vi "HFRR ADV v10.vi"() -> ()   [LabVIEW 2025] (continued)
                  n3633 = property on="Select Printer 3" class="DigNum (strict)"("Caption.Text"=w4909) -> ()  [unwired: 2 in, 2 out]
                }
                frame 116 {
                  n3634 = property on="Print" class="Bool (strict)"("Boolean Text.Text"=w4910) -> ()  [unwired: 2 in, 2 out]
                }
                frame 117 {
                  "String 41" <- w4911
                }
                frame 118 {
                  n3635 = property on="tested by" class="Str"("Caption.Text"=w4912) -> ()  [unwired: 2 in, 2 out]
                }
                frame 119 {
                }
                frame 120 {
                  n3636 = property on="Export" class="Bool (strict)"("Boolean Text.Text"=w4913) -> ()  [unwired: 2 in, 2 out]
                }
                frame 121 {
                  n3637 = property on="TEMP INTERCEPT:" class="DigNum (strict)"("Caption.Text"=w4914) -> ()  [unwired: 2 in, 2 out]
                }
                frame 122 {
                  n3638 = property on="AIR TEMP INTERCEPT:" class="DigNum (strict)"("Caption.Text"=w4915) -> ()  [unwired: 2 in, 2 out]
                }
                frame 123 {
                  n3639 = property on="Select File Type" class="Enum (strict)"("Caption.Text"=w4916) -> ()  [unwired: 2 in, 2 out]
                }
                frame 124 {
                  n3640 = property on="s.NO" class="Str"("Caption.Text"=w4917) -> ()  [unwired: 2 in, 2 out]
                  "String 45" <- w4917
                }
                frame 125 {
                  n3641 = property on="trip1 8" class="Bool (strict)"("Boolean Text.Text"=w4918) -> ()  [unwired: 2 in, 2 out]
                }
                frame 126, Default {
                }
              }
            }
          }
          frame #1 {
            w4926 = TRUE ("Visible")
            n3642 = local read "S 91"() -> (w4943:string)
            n3643 = local read "S 90"() -> (w4942:string)
            n3644 = local read "S 88"() -> (w4941:string)
            n3645 = property on="Threshold" class="DigNum (strict)"("Caption.Text"=w4943) -> ()  [unwired: 2 in, 2 out]
            n3646 = property on="File Path" class="Path"("Caption.Text"=w4942) -> ()  [unwired: 2 in, 2 out]
            n3647 = property on="SrvM CP" class="Bool (strict)"("Boolean Text.Text"=w4941) -> ()  [unwired: 2 in, 2 out]
            n3648 = local read "S 71"() -> (w4936:string)
            n3649 = local read "S 86"() -> (w4938:string)
            n3650 = local read "S 85"() -> (w4939:string)
            n3651 = local read "S 87"() -> (w4937:string)
            n3652 = local read "S 84"() -> (w4940:string)
            n3653 = local read "S 103"() -> (w4925:string)
            n3654 = local read "S 104"() -> (w4924:string)
            n3655 = property on="ENTER THE NEW PASSWORD" class="Str"("Caption.Text"=w4937) -> ()  [unwired: 2 in, 2 out]
            n3656 = property on="Password" class="Str"("Caption.Text"=w4939) -> ()  [unwired: 2 in, 2 out]
            n3657 = property on="ENTER CURRENT PASSWORD" class="Str"("Caption.Text"=w4938) -> ()  [unwired: 2 in, 2 out]
            n3658 = property on="EDIT" class="Bool (strict)"("Boolean Text.Text"=w4936) -> ()  [unwired: 2 in, 2 out]
            n3659 = property on="SAVE" class="Bool (strict)"("Boolean Text.Text"=w4940) -> ()  [unwired: 2 in, 2 out]
            n3660 = Build Array(w4925, w4924) -> (w4923:string[])
            n3661 = property on="Heater Button" class="Bool (strict)"("Strings [4]"=w4923) -> ()  [unwired: 2 in, 2 out]
            n3662 = property on="CH-HUMIDITY WET" class="DigNum (strict)"("Caption.Size to Text?"=w4926) -> ()  [unwired: 2 in, 2 out]
            n3663 = property on="CH-HUMIDITY DRY" class="DigNum (strict)"("Caption.Size to Text?"=w4926) -> ()  [unwired: 2 in, 2 out]
            n3664 = property on="CH-POWER -" class="DigNum (strict)"("Caption.Size to Text?"=w4926) -> ()  [unwired: 2 in, 2 out]
            n3665 = property on="CH-HEATER" class="DigNum (strict)"("Caption.Size to Text?"=w4926) -> ()  [unwired: 2 in, 2 out]
            n3666 = property on="CH-POWER +" class="DigNum (strict)"("Caption.Size to Text?"=w4926) -> ()  [unwired: 2 in, 2 out]
            n3667 = local read "S 92"() -> (w4935:string)
            n3668 = local read "S 93"() -> (w4934:string)
            n3669 = local read "S 105"() -> (w4921:string)
            n3670 = local read "S 106"() -> (w4920:string)
            n3671 = Build Array(w4935, w4934) -> ()  [unwired: 1 out]
            n3672 = Build Array(w4921, w4920) -> (w4922:string[])
            n3673 = local read "S 95"() -> (w4932:string)
            n3674 = local read "S 94"() -> (w4933:string)
            n3675 = local read "bs"() -> (w4948:string)
            n3676 = local read "as"() -> (w4949:string)
            n3677 = property on="Humidity" class="Bool (strict)"("Strings [4]"=w4922) -> ()  [unwired: 2 in, 2 out]
            n3678 = Concatenate Strings(w4948, "\r", w4949) -> ()  [unwired: 1 out]
            n3679 = property on="STROKE GAIN :" class="DigNum (strict)"("Caption.Text"=w4932) -> ()  [unwired: 2 in, 2 out]
            n3680 = property on="DISPLACEMENT :" class="DigNum (strict)"("Caption.Text"=w4933) -> ()  [unwired: 2 in, 2 out]
            n3681 = property on="Rh After" class="DigNum (strict)"("Caption.Size to Text?"=TRUE ("Caption.Size to Text")) -> ()  [unwired: 2 in, 2 out]
            n3682 = local read "S 48"() -> (w4972:string)
            n3683 = local read "S 50"() -> (w4970:string)
            n3684 = local read "S 51"() -> (w4969:string)
            n3685 = local read "S 49"() -> (w4971:string)
            n3686 = local read "S 52"() -> (w4968:string)
            n3687 = local read "as"() -> (w4953:string)
            n3688 = local read "bs"() -> (w4954:string)
            n3689 = local read "S 56"() -> (w4967:string)
            n3690 = local read "S 57"() -> (w4966:string)
            n3691 = local read "S 58"() -> (w4965:string)
            n3692 = local read "S 59"() -> (w4964:string)
            n3693 = property on="OPEN" class="Bool (strict)"("Boolean Text.Text"=w4968) -> ()  [unwired: 2 in, 2 out]
            n3694 = property on="OPEN 1" class="Bool (strict)"("Boolean Text.Text"=w4972) -> ()  [unwired: 2 in, 2 out]
            n3695 = property on="OPEN 2" class="Bool (strict)"("Boolean Text.Text"=w4971) -> ()  [unwired: 2 in, 2 out]
            n3696 = property on="OPEN 3" class="Bool (strict)"("Boolean Text.Text"=w4970) -> ()  [unwired: 2 in, 2 out]
            n3697 = property on="OPEN 4" class="Bool (strict)"("Boolean Text.Text"=w4969) -> ()  [unwired: 2 in, 2 out]
            n3698 = Concatenate Strings(w4954, "\r", w4953) -> ()  [unwired: 1 out]
            n3699 = local read "S 102"() -> (w4927:string)
            n3700 = property on="КОФ1" class="DigNum (strict)"("Caption.Text"=w4967) -> ()  [unwired: 2 in, 2 out]
            n3701 = local read "S 98"() -> (w4931:string)
            n3702 = local read "S 99"() -> (w4930:string)
            n3703 = local read "S 100"() -> (w4929:string)
            n3704 = local read "S 101"() -> (w4928:string)
            n3705 = property on="КОФ2" class="DigNum (strict)"("Caption.Text"=w4966) -> ()  [unwired: 2 in, 2 out]
            n3706 = property on="КОФ3" class="DigNum (strict)"("Caption.Text"=w4965) -> ()  [unwired: 2 in, 2 out]
            n3707 = property on="КОФ4" class="DigNum (strict)"("Caption.Text"=w4964) -> ()  [unwired: 2 in, 2 out]
            n3708 = local read "bs"() -> (w4952:string)
            n3709 = local read "as"() -> (w4951:string)
            n3710 = property on="CH-POWER +" class="DigNum (strict)"("Caption.Text"=w4931) -> ()  [unwired: 2 in, 2 out]
            n3711 = property on="CH-POWER -" class="DigNum (strict)"("Caption.Text"=w4930) -> ()  [unwired: 2 in, 2 out]
            n3712 = property on="CH-HEATER" class="DigNum (strict)"("Caption.Text"=w4929) -> ()  [unwired: 2 in, 2 out]
            n3713 = property on="CH-HUMIDITY DRY" class="DigNum (strict)"("Caption.Text"=w4928) -> ()  [unwired: 2 in, 2 out]
            n3714 = property on="CH-HUMIDITY WET" class="DigNum (strict)"("Caption.Text"=w4927) -> ()  [unwired: 2 in, 2 out]
            n3715 = local read "S 60"() -> (w4963:string)
            n3716 = local read "S 54"() -> (w4973:string)
            n3717 = Concatenate Strings(w4952, "\r", w4951) -> ()  [unwired: 1 out]
            n3718 = Concatenate Strings(w4973, w4963) -> ()  [unwired: 1 out]
            n3719 = local read "S 77"() -> (→"String 43":string)
            n3720 = local read "S 76"() -> (w4946:string)
            n3721 = local read "S 78"() -> (w4945:string)
            n3722 = local read "S 71"() -> (w4957:string)
            n3723 = local read "S 66"() -> (w4962:string)
            n3724 = local read "S 67"() -> (w4961:string)
            n3725 = local read "S 68"() -> (w4960:string)
            n3726 = local read "S 69"() -> (w4959:string)
            n3727 = local read "S 70"() -> (w4958:string)
            n3728 = property on="AIR TEMP" class="DigNum (strict)"("Caption.Text"=w4945) -> ()  [unwired: 2 in, 2 out]
            n3729 = property on="Set Strk" class="DigNum (strict)"("Caption.Text"=w4946) -> ()  [unwired: 2 in, 2 out]
            n3730 = property on="FRIC. FORCE :" class="DigNum (strict)"("Caption.Text"=w4962) -> ()  [unwired: 2 in, 2 out]
            n3731 = property on="TEMPERATURE :" class="DigNum (strict)"("Caption.Text"=w4961) -> ()  [unwired: 2 in, 2 out]
            n3732 = property on="SPEED OUT:" class="DigNum (strict)"("Caption.Text"=w4960) -> ()  [unwired: 2 in, 2 out]
            n3733 = property on="AIR TEMPERATURE :" class="DigNum (strict)"("Caption.Text"=w4959) -> ()  [unwired: 2 in, 2 out]
            n3734 = property on="HUMIDITY:" class="DigNum (strict)"("Caption.Text"=w4958) -> ()  [unwired: 2 in, 2 out]
            n3735 = property on="EDIT" class="Bool (strict)"("Boolean Text.Text"=w4957) -> ()  [unwired: 2 in, 2 out]
            n3736 = local read "S 79"() -> (w4944:string)
            n3737 = property on="Stroke" class="DigNum (strict)"("Caption.Text"=w4944) -> ()  [unwired: 2 in, 2 out]
          }
          frame #2 {
          }
        }
        n3738 = local write "Lan flag"(10.0 ("Lan flag")) -> ()
      }
      frame Enabled {
      }
    }
    n3739 = Wait (ms)(milliseconds to wait=u32 2000) -> ()  [unwired: 1 out]
    n3740 = local read "Quit"() -> (w4746:bool)
  }
  n3741 = disable-structure shown="Disabled" {
    frame Disabled {
      n3742 = while {
        tunnel: [w4975] -> _
        i -> [w4975]
        stop <- w4974 continue-if-true
        n3743 = Wait (ms)(milliseconds to wait=u32 50) -> ()  [unwired: 1 out]
        n3744 = stacked-sequence {
          frame #0 {
            # "Controls Text color"
            # "Controls BG color"
            n3745 = property on="FILE" class="Str"("Text.Text Colors:Text Color"="SC  Text") -> ()  [unwired: 2 in, 2 out]
            n3746 = property on="Fuel Discription :" class="Str"("Text.Text Colors:Text Color"="SC  Text") -> ()  [unwired: 2 in, 2 out]
            n3747 = property on="tested by" class="Str"("Text.Text Colors:Text Color"="SC  Text") -> ()  [unwired: 2 in, 2 out]
            n3748 = property on="Remarks :" class="Str"("Text.Text Colors:Text Color"="SC  Text") -> ()  [unwired: 2 in, 2 out]
            n3749 = property class="DigNum (strict)"("Numeric Text.Text Colors:BG Color"="NC BG") -> ()  [unwired: 2 in, 2 out]
            n3750 = property class="DigNum (strict)"("Numeric Text.Text Colors:BG Color"="NC BG") -> ()  [unwired: 2 in, 2 out]
            n3751 = property class="DigNum (strict)"("Numeric Text.Text Colors:BG Color"="NC BG") -> ()  [unwired: 2 in, 2 out]
            n3752 = property class="DigNum (strict)"("Numeric Text.Text Colors:BG Color"="NC BG") -> ()  [unwired: 2 in, 2 out]
            n3753 = property class="DigNum (strict)"("Numeric Text.Text Colors:BG Color"="NC BG") -> ()  [unwired: 2 in, 2 out]
            n3754 = property class="DigNum (strict)"("Numeric Text.Text Colors:BG Color"="NC BG") -> ()  [unwired: 2 in, 2 out]
            n3755 = property class="DigNum (strict)"("Numeric Text.Text Colors:BG Color"="NC BG") -> ()  [unwired: 2 in, 2 out]
            n3756 = property class="DigNum (strict)"("Numeric Text.Text Colors:BG Color"="NC BG") -> ()  [unwired: 2 in, 2 out]
            n3757 = property class="DigNum (strict)"("Numeric Text.Text Colors:BG Color"="NC BG") -> ()  [unwired: 2 in, 2 out]
            n3758 = property class="DigNum (strict)"("Numeric Text.Text Colors:BG Color"="NC BG") -> ()  [unwired: 2 in, 2 out]
            n3759 = property class="DigNum (strict)"("Numeric Text.Text Colors:BG Color"="NC BG") -> ()  [unwired: 2 in, 2 out]
            n3760 = property class="DigNum (strict)"("Numeric Text.Text Colors:BG Color"="NC BG") -> ()  [unwired: 2 in, 2 out]
            n3761 = property on="FILE" class="Str"("Text.Text Colors:BG Color"="SC BG 3") -> ()  [unwired: 2 in, 2 out]
            n3762 = property on="Fuel Discription :" class="Str"("Text.Text Colors:BG Color"="SC BG 3") -> ()  [unwired: 2 in, 2 out]
            n3763 = property on="tested by" class="Str"("Text.Text Colors:BG Color"="SC BG 3") -> ()  [unwired: 2 in, 2 out]
            n3764 = property on="Remarks :" class="Str"("Text.Text Colors:BG Color"="SC BG 3") -> ()  [unwired: 2 in, 2 out]
            n3765 = property class="DigNum (strict)"("Numeric Text.Text Colors:Text Color"="NC Text") -> ()  [unwired: 2 in, 2 out]
            n3766 = property class="DigNum (strict)"("Numeric Text.Text Colors:Text Color"="NC Text") -> ()  [unwired: 2 in, 2 out]
            n3767 = property class="DigNum (strict)"("Numeric Text.Text Colors:Text Color"="NC Text") -> ()  [unwired: 2 in, 2 out]
            n3768 = property class="DigNum (strict)"("Numeric Text.Text Colors:Text Color"="NC Text") -> ()  [unwired: 2 in, 2 out]
            n3769 = property class="DigNum (strict)"("Numeric Text.Text Colors:Text Color"="NC Text") -> ()  [unwired: 2 in, 2 out]
            n3770 = property class="DigNum (strict)"("Numeric Text.Text Colors:Text Color"="NC Text") -> ()  [unwired: 2 in, 2 out]
            n3771 = property class="DigNum (strict)"("Numeric Text.Text Colors:Text Color"="NC Text") -> ()  [unwired: 2 in, 2 out]
            n3772 = property class="DigNum (strict)"("Numeric Text.Text Colors:Text Color"="NC Text") -> ()  [unwired: 2 in, 2 out]
            n3773 = property class="DigNum (strict)"("Numeric Text.Text Colors:Text Color"="NC Text") -> ()  [unwired: 2 in, 2 out]
            n3774 = property class="DigNum (strict)"("Numeric Text.Text Colors:Text Color"="NC Text") -> ()  [unwired: 2 in, 2 out]
            n3775 = property class="DigNum (strict)"("Numeric Text.Text Colors:Text Color"="NC Text") -> ()  [unwired: 2 in, 2 out]
            n3776 = property class="DigNum (strict)"("Numeric Text.Text Colors:Text Color"="NC Text") -> ()  [unwired: 2 in, 2 out]
            n3777 = property class="DigNum (strict)"("Numeric Text.Text Colors:Text Color"="NI Text  2") -> ()  [unwired: 2 in, 2 out]
            n3778 = property class="DigNum (strict)"("Numeric Text.Text Colors:Text Color"="NI Text  2") -> ()  [unwired: 2 in, 2 out]
            n3779 = property class="DigNum (strict)"("Numeric Text.Text Colors:Text Color"="NI Text  2") -> ()  [unwired: 2 in, 2 out]
            n3780 = property class="DigNum (strict)"("Numeric Text.Text Colors:Text Color"="NI Text  2") -> ()  [unwired: 2 in, 2 out]
            n3781 = property class="DigNum (strict)"("Numeric Text.Text Colors:Text Color"="NI Text  2") -> ()  [unwired: 2 in, 2 out]
            n3782 = property class="DigNum (strict)"("Numeric Text.Text Colors:Text Color"="NI Text  2") -> ()  [unwired: 2 in, 2 out]
            n3783 = property class="DigNum (strict)"("Numeric Text.Text Colors:Text Color"="NI Text  2") -> ()  [unwired: 2 in, 2 out]
            n3784 = property class="DigNum (strict)"("Numeric Text.Text Colors:Text Color"="NI Text  2") -> ()  [unwired: 2 in, 2 out]
            n3785 = property class="DigNum (strict)"("Numeric Text.Text Colors:Text Color"="NI Text  2") -> ()  [unwired: 2 in, 2 out]
            n3786 = property class="DigNum (strict)"("Numeric Text.Text Colors:Text Color"="NI Text  2") -> ()  [unwired: 2 in, 2 out]
            n3787 = property class="DigNum (strict)"("Numeric Text.Text Colors:Text Color"="NI Text  2") -> ()  [unwired: 2 in, 2 out]
            n3788 = property class="DigNum (strict)"("Numeric Text.Text Colors:Text Color"="NI Text  2") -> ()  [unwired: 2 in, 2 out]
            n3789 = property class="DigNum (strict)"("Numeric Text.Text Colors:Text Color"="NI Text  2") -> ()  [unwired: 2 in, 2 out]
            n3790 = property class="DigNum (strict)"("Numeric Text.Text Colors:Text Color"="NI Text  2") -> ()  [unwired: 2 in, 2 out]
            n3791 = property class="DigNum (strict)"("Numeric Text.Text Colors:Text Color"="NI Text  2") -> ()  [unwired: 2 in, 2 out]
            n3792 = property class="DigNum (strict)"("Numeric Text.Text Colors:Text Color"="NI Text  2") -> ()  [unwired: 2 in, 2 out]
            n3793 = property on="Coefficient Of Friction" class="XYGraph (strict)"("Plot Area:Colors:FG Color"="GFG  2", "Plot Area:Colors:BG Color"="GBG   2") -> ()  [unwired: 2 in, 2 out]
            n3794 = property on="Humidity ( %RH )" class="XYGraph (strict)"("Plot Area:Colors:FG Color"="GFG  2", "Plot Area:Colors:BG Color"="GBG   2") -> ()  [unwired: 2 in, 2 out]
            n3795 = property on="Air Temperature  ( °C )" class="XYGraph (strict)"("Plot Area:Colors:FG Color"="GFG  2", "Plot Area:Colors:BG Color"="GBG   2") -> ()  [unwired: 2 in, 2 out]
            n3796 = property on="Sample Temperature ( °C )" class="XYGraph (strict)"("Plot Area:Colors:FG Color"="GFG  2", "Plot Area:Colors:BG Color"="GBG   2") -> ()  [unwired: 2 in, 2 out]
            n3797 = property class="DigNum (strict)"("Numeric Text.Text Colors:BG Color"="NI BG 2") -> ()  [unwired: 2 in, 2 out]
            n3798 = property class="DigNum (strict)"("Numeric Text.Text Colors:BG Color"="NI BG 2") -> ()  [unwired: 2 in, 2 out]
            n3799 = property class="DigNum (strict)"("Numeric Text.Text Colors:BG Color"="NI BG 2") -> ()  [unwired: 2 in, 2 out]
            n3800 = property class="DigNum (strict)"("Numeric Text.Text Colors:BG Color"="NI BG 2") -> ()  [unwired: 2 in, 2 out]
            n3801 = property class="DigNum (strict)"("Numeric Text.Text Colors:BG Color"="NI BG 2") -> ()  [unwired: 2 in, 2 out]
            n3802 = property class="DigNum (strict)"("Numeric Text.Text Colors:BG Color"="NI BG 2") -> ()  [unwired: 2 in, 2 out]
            n3803 = property class="DigNum (strict)"("Numeric Text.Text Colors:BG Color"="NI BG 2") -> ()  [unwired: 2 in, 2 out]
            n3804 = property class="DigNum (strict)"("Numeric Text.Text Colors:BG Color"="NI BG 2") -> ()  [unwired: 2 in, 2 out]
            n3805 = property class="DigNum (strict)"("Numeric Text.Text Colors:BG Color"="NI BG 2") -> ()  [unwired: 2 in, 2 out]
            n3806 = property class="DigNum (strict)"("Numeric Text.Text Colors:BG Color"="NI BG 2") -> ()  [unwired: 2 in, 2 out]
            n3807 = property class="DigNum (strict)"("Numeric Text.Text Colors:BG Color"="NI BG 2") -> ()  [unwired: 2 in, 2 out]
            n3808 = property class="DigNum (strict)"("Numeric Text.Text Colors:BG Color"="NI BG 2") -> ()  [unwired: 2 in, 2 out]
            n3809 = property class="DigNum (strict)"("Numeric Text.Text Colors:BG Color"="NI BG 2") -> ()  [unwired: 2 in, 2 out]
            n3810 = property class="DigNum (strict)"("Numeric Text.Text Colors:BG Color"="NI BG 2") -> ()  [unwired: 2 in, 2 out]
            n3811 = property class="DigNum (strict)"("Numeric Text.Text Colors:BG Color"="NI BG 2") -> ()  [unwired: 2 in, 2 out]
            n3812 = property class="DigNum (strict)"("Numeric Text.Text Colors:BG Color"="NI BG 2") -> ()  [unwired: 2 in, 2 out]
            n3813 = property class="Bool"("Colors [4]"="Boolean BC T & BG") -> ()  [unwired: 2 in, 2 out]
            n3814 = property on="Save & Continue" class="Bool (strict)"("Colors [4]"="Boolean BC T & BG") -> ()  [unwired: 2 in, 2 out]
            n3815 = property on="Heater Button" class="Bool (strict)"("Colors [4]"="Boolean BC T & BG") -> ()  [unwired: 2 in, 2 out]
            n3816 = property class="Bool"("Colors [4]"="Boolean BC T & BG") -> ()  [unwired: 2 in, 2 out]
            n3817 = property on="Humidity" class="Bool (strict)"("Colors [4]"="Boolean BC T & BG") -> ()  [unwired: 2 in, 2 out]
            n3818 = property class="Bool (strict)"("Colors [4]"="Boolean BC T & BG") -> ()  [unwired: 2 in, 2 out]
            n3819 = property on="RUN" class="Bool (strict)"("Colors [4]"="Boolean BC T & BG") -> ()  [unwired: 2 in, 2 out]
            n3820 = property on="trip1 8" class="Bool (strict)"("Colors [4]"="Boolean BC T & BG") -> ()  [unwired: 2 in, 2 out]
            n3821 = property class="Bool"("Colors [4]"="Boolean BC T & BG") -> ()  [unwired: 2 in, 2 out]
            n3822 = property class="Bool (strict)"("Colors [4]"="Boolean BC T & BG") -> ()  [unwired: 2 in, 2 out]
            n3823 = property on="OPEN 1" class="Bool (strict)"("Colors [4]"="Boolean BC T & BG 2") -> ()  [unwired: 2 in, 2 out]
            n3824 = property on="OPEN 2" class="Bool (strict)"("Colors [4]"="Boolean BC T & BG 2") -> ()  [unwired: 2 in, 2 out]
            n3825 = property on="OPEN 3" class="Bool (strict)"("Colors [4]"="Boolean BC T & BG 2") -> ()  [unwired: 2 in, 2 out]
            n3826 = property on="OPEN 4" class="Bool (strict)"("Colors [4]"="Boolean BC T & BG 2") -> ()  [unwired: 2 in, 2 out]
            n3827 = property on="OPEN" class="Bool (strict)"("Colors [4]"="Boolean BC T & BG 2") -> ()  [unwired: 2 in, 2 out]
            n3828 = property on="rstv2" class="Bool"("Colors [4]"="Boolean BC T & BG 2") -> ()  [unwired: 2 in, 2 out]
            n3829 = property on="RST CP" class="Bool"("Colors [4]"="Boolean BC T & BG 2") -> ()  [unwired: 2 in, 2 out]
            n3830 = property on="RSTV1 3" class="Bool"("Colors [4]"="Boolean BC T & BG 2") -> ()  [unwired: 2 in, 2 out]
            n3831 = property on="RSTV1 2" class="Bool"("Colors [4]"="Boolean BC T & BG 2") -> ()  [unwired: 2 in, 2 out]
          }
          frame #1 {
          }
        }
        n3832 = local read "Quit"() -> (w4974:bool)
      }
    }
    frame Enabled {
    }
  }
  n3833 = while {
    shift-right: [w4992] -> _
    shift-left: _ -> [w4993]
    shift-right: [w4990] -> _
    shift-left: T17 {"Read Heave and Surge"="", "Bytes at Heave Port"=0.0, "Heave and Surge COM Port:"="COM9", "Com Port 2"="COM7", "Residual Due"="", "Heave COM Status 2"=TRUE, "Heave COM Status"=TRUE, "Port 2"=TRUE, "Sway PPR"=6400.0, "Surge PPR"=6400.0, "Heave PPR"=6400.0, "Sway Pitch"=2.0, "Surge Pitch"=3.0, "Heave Pitch"=4.0, "Sway Pulses/mm"=320.0, "Surge Pulses/mm"=1600.0, "Heave Pulses/mm"=1600.0, "inner loop"=0.0, "Read Heave and Surge 2"="", "String 36"="", "Write S"=FALSE, "WriteCC1"=[""], "Heave COM Loop"=0, "LastCom"="", "EXIT"=FALSE, "Error Heave"={"status"=TRUE, "code"=-1073807343, "source"=""}} -> [w4989]
    shift-right: [w4987] -> _
    shift-left: enum16{"init", "MAIN", "Panel Close"}."init" -> [w4988]
    stop <- w4991 stop-if-true
    n3834 = case shown="\"init\"" w4988 {
      tunnel: w4993 -> [w5007 w5022 w5092 w5094]
      tunnel: [w5001 w5040 w5092 w5094] -> w4992
      tunnel: [_ _ TRUE _] -> w4991
      tunnel: [w4997 w5037 w5090 w5093] -> w4990
      tunnel: w4989 -> [w5004 w5021 w5090 w5093]
      tunnel: [enum16{"init", "MAIN", "Panel Close"}."MAIN" w5015 _ _] -> w4987
      frame "init" {
        n3835 = Bundle By Name(cluster=w5004, "Heave and Surge COM Port:"="C3 :") -> (w5003:T17)
        n3836 = call "Instrument fgv.vi"("Enum"=T27."INIT", "error in (no error) 2"=w5007, "INPUT"=w5003) -> ("error"=w5005:errorcluster, "output"=w5000:T17)  [unwired: 6 in, 1 out]
        n3837 = case shown="No Error" w5005 {
          selector: w5005 -> [w5009 _]
          tunnel: [w5009 w5013] -> w5001
          tunnel: w5000 -> [w5008 w5011]
          tunnel: [w5008 w5010] -> w4998
          frame No Error {
          }
          frame Error {
            n3838 = call "Instrument fgv.vi"("Enum"=T27."ERROR INIT", "INPUT"=w5011) -> ("error"=w5014:errorcluster, "output"=w5010:T17)  [unwired: 7 in, 1 out]
            n3839 = call <vilib>:"Clear Errors.vi"("error in (no error)"=w5014) -> ("error out"=w5013:errorcluster)  [unwired: 5 in, 1 out]
          }
        }
        n3840 = local read "LastCom"() -> (w4996:string)
        n3841 = Unbundle By Name(w4998) -> ("Heave COM Status 2"=→"COM Status" →"Instrument Status":bool, "Error Heave"=→"Error":errorcluster)  [unwired: 1 out]
        n3842 = Bundle By Name(cluster=w4998, "LastCom"=w4996) -> (w4997:T17)
      }
      frame "MAIN" {
        n3843 = Unbundle By Name(w5021) -> ("Com Port 2"=w5042:refnum<visa-resource-name>)
        n3844 = local write "Com Port 4"(w5042) -> ()
        n3845 = local read "C3 :"() -> (w5019:refnum<visa-resource-name>)
        n3846 = Divide(x="Heave PPR", y="Heave Pitch") -> (x/y=→"Heave Pulses/mm":dbl)
        n3847 = Bundle By Name(cluster=w5021, "Heave and Surge COM Port:"=w5019) -> (w5020:T17)
        n3848 = Equal?(x=w5042, y=w5019) -> (x = y?=w5041:bool)
        n3849 = Divide(x="Sway PPR", y="Sway Pitch") -> (x/y=→"Sway Pulses/mm":dbl)
        n3850 = case shown="False" w5041 {
          tunnel: [w5046 w5063] -> w5040
          tunnel: w5022 -> [w5047 w5069]
          tunnel: w5020 -> [w5045 w5067]
          tunnel: [w5044 w5062] -> w5037
          frame False {
            n3851 = call <vilib>:"Clear Errors.vi"("error in (no error)"=w5047) -> ("error out"=w5043:errorcluster)  [unwired: 5 in, 1 out]
            n3852 = call "Instrument fgv.vi"("Enum"=T27."ERROR INIT", "error in (no error) 2"=w5043, "INPUT"=w5045) -> ("error"=w5049:errorcluster, "output"=w5044:T17)  [unwired: 6 in, 1 out]
            n3853 = call <vilib>:"Clear Errors.vi"("error in (no error)"=w5049) -> ("error out"=w5046:errorcluster)  [unwired: 5 in, 1 out]
          }
          frame True {
            n3854 = call "Instrument fgv.vi"("Enum"=T27."READ", "error in (no error) 2"=w5069, "INPUT"=w5067) -> ("error"=w5068:errorcluster, "output"=w5059:T17)  [unwired: 6 in, 1 out]
            n3855 = Bundle By Name(cluster=w5059, "String 36"="String 11") -> (w5058:T17)
            n3856 = case shown="True" "Write S" {
              selector: "Write S" -> [_ w5089]
              tunnel: w5068 -> [w5082 w5088]
              tunnel: [w5082 w5087] -> w5055
              tunnel: w5058 -> [w5081 w5084]
              tunnel: [w5081 w5083] -> w5054
              frame False {
              }
              frame True {
                n3857 = Not(x=w5089) -> (.not. x?=w5085:bool)
                n3858 = local write "Write S"(w5085) -> ()
                n3859 = call "Instrument fgv.vi"("Enum"=T27."MANUAL WRITE", "error in (no error) 2"=w5088, "INPUT"=w5084) -> ("error"=w5087:errorcluster, "output"=w5083:T17)  [unwired: 6 in, 1 out]
              }
            }
            n3860 = Array Size(array="WriteHumidity") -> (size(s)=w5052:i32)
            n3861 = Greater Than 0?(x=w5052) -> (x > 0?=w5050:bool)
            n3862 = call "Instrument fgv.vi"("Enum"=T27."WRITE", "error in (no error) 2"=w5055, "WriteCC1"="WriteHumidity", "INPUT"=w5054) -> ("error"=w5065:errorcluster, "WriteCC1 2"=w5053:string[], "output"=w5064:T17)  [unwired: 5 in]
            n3863 = case shown="True" w5050 {
              tunnel: w5053 -> [_ w5071]
              frame False {
              }
              frame True {
                n3864 = local write "WriteHumidity"(w5071) -> ()
              }
            }
            n3865 = case shown="Error" w5065 {
              selector: w5065 -> [w5072 w5075]
              tunnel: w5064 -> [w5073 w5080]
              tunnel: [w5073 w5079] -> w5062
              tunnel: [w5072 w5077] -> w5063
              frame No Error {
              }
              frame Error {
                n3866 = call <vilib>:"Clear Errors.vi"("error in (no error)"=w5075) -> ("error out"=w5074:errorcluster)  [unwired: 5 in, 1 out]
                n3867 = call "Instrument fgv.vi"("Enum"=T27."ERROR INIT", "error in (no error) 2"=w5074, "INPUT"=w5080) -> ("error"=w5078:errorcluster, "output"=w5079:T17)  [unwired: 6 in, 1 out]
                n3868 = call <vilib>:"Clear Errors.vi"("error in (no error)"=w5078) -> ("error out"=w5077:errorcluster)  [unwired: 5 in, 1 out]
              }
            }
            n3869 = Unbundle By Name(w5062) -> ("LastCom"=→"LastCom":string, "Read Heave and Surge"=→"Read Humidity":string)
          }
        }
        n3870 = Divide(x="Surge PPR", y="Surge Pitch") -> (x/y=→"Surge Pulses/mm":dbl)
        n3871 = Unbundle By Name(w5037) -> ("Heave COM Status 2"=w5039:bool, "Heave COM Status"=w5038:bool, "Error Heave"=w5035:errorcluster, "Bytes at Heave Port"=→"Bytes at Humidity Port":dbl)
        n3872 = Unbundle By Name(w5035) -> ("status"=→"Humidity Port":bool)
        n3873 = Not(x=w5038) -> (.not. x?=w5023:bool)
        n3874 = local write "Error"(w5035) -> ()
        n3875 = Not(x=w5039) -> (.not. x?=w5024:bool)
        n3876 = local write "Instrument Status"(w5023) -> ()
        n3877 = local write "COM Status"(w5024) -> ()
        n3878 = local read "Quit"() -> (w5016:bool)
        n3879 = Select(t=enum16{"init", "MAIN", "Panel Close"}."Panel Close", s=w5016, f=enum16{"init", "MAIN", "Panel Close"}."MAIN") -> (s? t:f=w5015:enum16{"init", "MAIN", "Panel Close"})
      }
      frame "Panel Close" {
      }
      frame Default {
      }
    }
  }
  n3880 = while {
    stop <- w5120 stop-if-true
    n3881 = local read "Read Humidity"() -> (w5101:string)
    n3882 = call <vilib>:"High Resolution Polling Wait.vi"("seconds to wait"=0.1) -> ()  [unwired: 10 in, 1 out]
    n3883 = Spreadsheet String To Array(delimiter (Tab)=",", format string="", spreadsheet string=w5101, array type (2D Dbl)=string[] []) -> (array=w5115:string[])
    n3884 = for {
      tunnel: w5115 -> [w5125] mode=indexing
      tunnel: string[] ["STATE;", "SET;", "RH;", "T;", "AMB_RH;", "AMB_T;", "PUMP;", "FAN_IN;", "FAN_OUT;", "DEHUM;", "CURRENT;", "STALL;"] -> [w5124] mode=indexing
      tunnel: [w5123] -> w5114 mode=indexing
      n3885 = Match Pattern(string=w5125, regular expression=w5124) -> (after substring=w5123:string)  [unwired: 1 in, 3 out]
    }
    n3886 = Index Array(array=w5114) -> (element #1=→"STATE :":string, element #2=→"SET :":string, element #3=w5103:string, element #4=→"T :":string, element #5=w5100:string, element #6=→"AMB_T :":string, element #7=→"PUMP :":string, element #8=→"FAN_IN :":string, element #9=→"FAN_OUT :":string, element #10=→"DEHUM :":string, element #11=→"CURRENT :":string, element #12=→"STALL :":string)  [unwired: 12 in]
    "RH :" <- w5103
    "AMB_RH :" <- w5100
    n3887 = Fract/Exp String To Number(string=w5103) -> (number=w5095:dbl)  [unwired: 3 in, 1 out]
    n3888 = Fract/Exp String To Number(string=w5100) -> (number=w5099:dbl)  [unwired: 3 in, 1 out]
    n3889 = local write "Ambient Humidity :"(w5099) -> ()
    n3890 = Equal?(x=w5095, y=0.0) -> (x = y?=w5097:bool)
    n3891 = case shown="True" w5097 {
      tunnel: [w5121 w5122] -> w5096
      tunnel: w5095 -> [w5121 _]
      frame False {
        (unwired) 0.0
        "Humidity temp" <- w5121
      }
      frame True {
        n3892 = local read "Humidity temp"() -> (w5122:dbl)
      }
    }
    "RH Numeric:" <- w5096
    n3893 = local read "Quit"() -> (w5120:bool)
  }
  n3894 = disable-structure shown="Disabled" {
    frame Disabled {
      n3895 = while {
        tunnel: [w5359] -> _
        i -> [w5359]
        stop <- w5356 stop-if-true
        n3896 = local read "powstat"() -> (w5357:bool)
        n3897 = case shown="True" w5357 {
          frame False {
          }
          frame True {
            n3898 = local read "RUN"() -> (w5360:bool)
            n3899 = case shown="True" w5360 {
              frame False {
                w5390 = 65.0 ("y")
                n3900 = local read "Set Hz"() -> (w5418:dbl)
                n3901 = local read "NORMAL LOAD"() -> (w5419:dbl)
                n3902 = Multiply(x=w5418, y=60.0) -> (x*y=w5425:dbl)
                n3903 = Multiply(x=1.2 ("y"), y=0.949) -> (x*y=w5394:dbl)
                n3904 = Multiply(x=1.2 ("y"), y=0.8166) -> (x*y=w5398:dbl)
                n3905 = Multiply(x=1.2 ("y"), y=0.851) -> (x*y=w5393:dbl)
                n3906 = local read "FF 2"() -> (w5417:dbl)
                n3907 = Absolute Value(x=w5425) -> (abs(x)=w5423:dbl)
                n3908 = local read "Stroke"() -> (w5392:dbl)
                n3909 = Less?(x=w5392, y=w5398) -> (x < y?=w5395:bool)
                n3910 = In Range and Coerce(upper limit=w5394, x=w5392, lower limit=w5393) -> (In Range?=w5396:bool)  [unwired: 1 out]
                n3911 = case shown="13.." w5417 {
                  tunnel: [1 2 3] -> w5415
                  frame 0..10, Default {
                    # "Normal"
                  }
                  frame 11, 12 {
                  }
                  frame 13.. {
                  }
                }
                "FF STATE" <- w5415
                n3912 = local read "TEMP"() -> (w5378:dbl)
                n3913 = case shown="3601.." w5423 {
                  tunnel: [1 2 3] -> w5421
                  frame 0..3000, Default {
                    # "Normal"
                  }
                  frame 3001..3600 {
                  }
                  frame 3601.. {
                  }
                }
                n3914 = case shown="11.." w5419 {
                  tunnel: [1 3] -> w5420
                  frame 1..10, Default {
                  }
                  frame 11.. {
                  }
                }
                "NL STATE" <- w5420
                n3915 = Multiply(x=1.2 ("y"), y=0.95) -> (x*y=w5408:dbl)
                n3916 = Multiply(x=w5390, y=0.954) -> (x*y=w5382:dbl)
                n3917 = Or(x=w5395, y=w5396) -> (x .or. y?=w5397:bool)
                n3918 = Greater Or Equal?(x=w5392, y=w5408) -> (x >= y?=w5405:bool)
                n3919 = Multiply(x=w5390, y=0.99) -> (x*y=w5379:dbl)
                n3920 = Greater Or Equal?(x=w5378, y=w5379) -> (x >= y?=w5384:bool)
                n3921 = Greater Or Equal?(x=w5378, y=w5382) -> (x >= y?=w5381:bool)
                n3922 = case shown="0, 1, Default" w5392 {
                  tunnel: [1 3] -> w5409
                  frame 0, 1, Default {
                  }
                  frame 2.. {
                  }
                }
                n3923 = case shown="True" w5405 {
                  tunnel: [1 3] -> w5410
                  frame False {
                  }
                  frame True {
                  }
                }
                n3924 = case shown="True" w5397 {
                  tunnel: [1 2] -> w5411
                  frame False {
                  }
                  frame True {
                  }
                }
                n3925 = case shown="..0" w5378 {
                  tunnel: [2 3 3 1] -> w5385
                  frame 61, 62 {
                  }
                  frame 63.. {
                  }
                  frame ..0 {
                  }
                  frame 10..60, Default {
                  }
                }
                n3926 = case shown="True" w5384 {
                  tunnel: [1 3] -> w5386
                  frame False {
                  }
                  frame True {
                  }
                }
                n3927 = Number To Decimal String(number=w5421) -> (decimal integer string=w5422:string)  [unwired: 1 in]
                n3928 = case shown="True" w5381 {
                  tunnel: [1 2] -> w5387
                  frame False {
                  }
                  frame True {
                  }
                }
                n3929 = Number To Decimal String(number=1) -> (decimal integer string=→"Air temp":string)  [unwired: 1 in]
                n3930 = Number To Decimal String(number=w5415) -> (decimal integer string=→"ff_st":string)  [unwired: 1 in]
                n3931 = local write "sp_st"(w5422) -> ()
                n3932 = Number To Decimal String(number=w5420) -> (decimal integer string=→"nl_st":string)  [unwired: 1 in]
                n3933 = Build Array(w5385, w5386, w5387) -> (w5388:i32[])
                n3934 = Build Array(w5409, w5410, w5411) -> (w5412:i32[])
                n3935 = Array Max & Min(array=w5388) -> (max value=w5389:i32)  [unwired: 3 out]
                n3936 = Array Max & Min(array=w5412) -> (max value=w5413:i32)  [unwired: 3 out]
                n3937 = Number To Decimal String(number=w5389) -> (decimal integer string=w5377:string)  [unwired: 1 in]
                n3938 = Number To Decimal String(number=w5413) -> (decimal integer string=→"Stroke Ln 2":string)  [unwired: 1 in]
                n3939 = local write "temp_st"(w5377) -> ()
              }
              frame True {
                w5475 = 65.0 ("y")
                # "Healthy -1\nWarning -2\nError -3"
                n3940 = local read "TEMP"() -> (w5486:dbl)
                n3941 = local read "NORMAL LOAD"() -> (w5490:dbl)
                n3942 = local read "Set Hz"() -> (w5488:dbl)
                n3943 = Multiply(x=1.2 ("y"), y=0.949) -> (x*y=w5470:dbl)
                n3944 = Multiply(x=1.2 ("y"), y=0.8166) -> (x*y=w5466:dbl)
                n3945 = Multiply(x=1.2 ("y"), y=0.851) -> (x*y=w5471:dbl)
                n3946 = Multiply(x=w5475, y=0.954) -> (x*y=w5482:dbl)
                n3947 = Multiply(x=w5475, y=0.99) -> (x*y=w5485:dbl)
                n3948 = Greater Or Equal?(x=w5486, y=w5485) -> (x >= y?=w5480:bool)
                n3949 = Multiply(x=w5488, y=60.0) -> (x*y=w5494:dbl)
                n3950 = Greater Or Equal?(x=w5486, y=w5482) -> (x >= y?=w5483:bool)
                n3951 = local read "FF 2"() -> (w5489:dbl)
                n3952 = local read "Stroke"() -> (w5472:dbl)
                n3953 = Less?(x=w5472, y=w5466) -> (x < y?=w5469:bool)
                n3954 = In Range and Coerce(upper limit=w5470, x=w5472, lower limit=w5471) -> (In Range?=w5468:bool)  [unwired: 1 out]
                n3955 = Absolute Value(x=w5494) -> (abs(x)=w5492:dbl)
                n3956 = case shown="63.." w5486 {
                  tunnel: [2 3 3 1] -> w5479
                  frame 61, 62 {
                  }
                  frame 63.. {
                  }
                  frame ..0 {
                  }
                  frame 10..60, Default {
                  }
                }
                n3957 = case shown="True" w5480 {
                  tunnel: [1 3] -> w5478
                  frame False {
                  }
                  frame True {
                  }
                }
                n3958 = case shown="True" w5483 {
                  tunnel: [1 2] -> w5477
                  frame False {
                  }
                  frame True {
                  }
                }
                n3959 = Multiply(x=1.2 ("y"), y=0.95) -> (x*y=w5456:dbl)
                n3960 = case shown="1..10, Default" w5490 {
                  tunnel: [1 3] -> w5497
                  frame 1..10, Default {
                  }
                  frame 11.. {
                  }
                }
                n3961 = case shown="0..10, Default" w5489 {
                  tunnel: [1 2 3] -> w5496
                  frame 0..10, Default {
                  }
                  frame 11, 12 {
                  }
                  frame 13.. {
                  }
                }
                n3962 = case shown="3601.." w5492 {
                  tunnel: [1 2 3] -> w5491
                  frame 0..3000, Default {
                    # "Normal"
                  }
                  frame 3001..3600 {
                  }
                  frame 3601.. {
                  }
                }
                n3963 = Or(x=w5469, y=w5468) -> (x .or. y?=w5467:bool)
                n3964 = Greater Or Equal?(x=w5472, y=w5456) -> (x >= y?=w5459:bool)
                n3965 = case shown="0, 1, Default" w5472 {
                  tunnel: [1 3] -> w5455
                  frame 0, 1, Default {
                  }
                  frame 2.. {
                  }
                }
                n3966 = case shown="True" w5459 {
                  tunnel: [1 3] -> w5454
                  frame False {
                  }
                  frame True {
                  }
                }
                n3967 = case shown="True" w5467 {
                  tunnel: [1 2] -> w5453
                  frame False {
                  }
                  frame True {
                  }
                }
                n3968 = Build Array(w5479, w5478, w5477) -> (w5476:i32[])
                n3969 = Number To Decimal String(number=w5491) -> (decimal integer string=→"sp_st":string)  [unwired: 1 in]
                n3970 = Array Max & Min(array=w5476) -> (max value=w5473:i32)  [unwired: 3 out]
                "TEMP STATE" <- w5473
                n3971 = Number To Decimal String(number=w5497) -> (decimal integer string=w5500:string)  [unwired: 1 in]
                n3972 = Number To Decimal String(number=w5496) -> (decimal integer string=w5498:string)  [unwired: 1 in]
                n3973 = Number To Decimal String(number=w5473) -> (decimal integer string=→"temp_st":string)  [unwired: 1 in]
                n3974 = Build Array(w5455, w5454, w5453) -> (w5452:i32[])
                n3975 = local write "nl_st"(w5500) -> ()
                n3976 = local write "ff_st"(w5498) -> ()
                n3977 = Number To Decimal String(number=1) -> (decimal integer string=w5495:string)  [unwired: 1 in]
                n3978 = Array Max & Min(array=w5452) -> (max value=w5451:i32)  [unwired: 3 out]
                n3979 = local write "Air temp"(w5495) -> ()
                n3980 = Number To Decimal String(number=w5451) -> (decimal integer string=w5450:string)  [unwired: 1 in]
                n3981 = local write "Stroke Ln 2"(w5450) -> ()
              }
            }
            n3982 = local read "Stroke Ln 2"() -> (w5362:string)
            n3983 = local read "nl_st"() -> (w5368:string)
            n3984 = local read "ff_st"() -> (w5365:string)
            n3985 = local read "sp_st"() -> (w5366:string)
            n3986 = local read "temp_st"() -> (w5367:string)
            n3987 = local read "Air temp"() -> (w5361:string)
            n3988 = Replace Array Subset(array="in", new element #1=w5368, index #1=1 ("index"), new element #2=w5365, index #2=2 ("index"), new element #3=w5367, index #3=3 ("index"), new element #4=w5366, index #4=4 ("index"), new element #5=w5362, index #5=5 ("index"), new element #6=w5361, index #6=6 ("index"), new element #7="Sensor State" ("new element/subarray"), index #7=0 ("index")) -> (→"out":string[])
          }
        }
        n3989 = Wait (ms)(milliseconds to wait=u32 10) -> ()  [unwired: 1 out]
        n3990 = local read "Quit"() -> (w5356:bool)
      }
      n3991 = while {
        stop <- w5331 stop-if-true
        n3992 = local read "run replace"() -> (w5333:bool)
        n3993 = Wait (ms)(milliseconds to wait=u32 100) -> ()  [unwired: 1 out]
        n3994 = Equal?(x="FLAG 2", y=0.0) -> (x = y?=w5334:bool)
        n3995 = case shown="True" w5334 {
          frame False {
          }
          frame True {
            n3996 = local write "FLAG 2"(100.0 ("FLAG 2")) -> ()
            n3997 = call <vilib>:"Read Characters From File.vi"("file path (dialog if empty)"=path "C:/LAB-IQ-NXT/WO 2449 TT.sig", "convert eol? (no:F)"=FALSE ("append to file? (new file:F)")) -> ("character string"=w5337:string)  [unwired: 4 in, 3 out]
            n3998 = call <vilib>:"Read Characters From File.vi"("file path (dialog if empty)"=path "C:/LAB-IQ-NXT/WO 2449 TRH.sig", "convert eol? (no:F)"=FALSE ("append to file? (new file:F)")) -> ("character string"=w5338:string)  [unwired: 4 in, 3 out]
            n3999 = Decimal String To Number(string=w5337) -> (number=w5339:i32)  [unwired: 2 in, 1 out]
            n4000 = local write "Total No. of Tests"(w5339) -> ()
            n4001 = Decimal String To Number(string=w5338) -> (number=w5342:i32)  [unwired: 2 in, 1 out]
            n4002 = local write "SEN.RUN HRS"(w5342) -> ()
          }
        }
        n4003 = case shown="True" w5333 {
          frame False {
          }
          frame True {
            n4004 = Equal?(x="FLAG 4", y=0.0) -> (x = y?=w5346:bool)
            n4005 = case shown="False" w5346 {
              frame False {
                n4006 = Get Date/Time In Seconds() -> (seconds since 1Jan1904=w5352:timestamp)
                n4007 = local read "START 3"() -> (w5350:dbl)
                n4008 = To Double Precision Float(number=w5352) -> (double precision float=w5351:dbl)
                n4009 = Subtract(x=w5351, y=w5350) -> (x-y=→"SENSOR TIME":dbl)
              }
              frame True {
                n4010 = Get Date/Time In Seconds() -> (seconds since 1Jan1904=w5354:timestamp)
                n4011 = local write "FLAG 4"(100.0 ("FLAG")) -> ()
                n4012 = To Double Precision Float(number=w5354) -> (double precision float=→"START 3":dbl)
              }
            }
          }
        }
        n4013 = local read "Quit"() -> (w5331:bool)
      }
      n4014 = while {
        shift-right: [w5131] -> _
        shift-left: _ -> [w5132]
        tunnel: [w5127] -> _
        i -> [w5127]
        stop <- w5126 stop-if-true
        n4015 = Wait (ms)(milliseconds to wait=u32 50 ("Refresh Rate (ms)")) -> ()  [unwired: 1 out]
        n4016 = local read "Json End Flg"() -> (w5128:bool)
        n4017 = Not(x="Upld AR 2") -> ()  [unwired: 1 out]
        n4018 = local read "Upld AR 2"() -> (w5129:bool)
        n4019 = call "Elapsed Time9"("Time Target (s)"="Sen.Upload Rate (s)", "Reset"=FALSE, "Auto Reset"=TRUE) -> ("Time has Elapsed"=w5138:bool)  [unwired: 9 in, 7 out]
        n4020 = Or(x=w5138, y=w5128) -> (x .or. y?=w5134:bool)
        n4021 = case shown="True" w5134 {
          frame False {
          }
          frame True {
            w5230 = "\"SensorName\":\"" ("string")
            w5200 = " \"},{"
            w5225 = "\",\"SensorState\":\""
            w5227 = "\",\"SensorModelNumber\":\"" ("string")
            w5226 = "\",\"SensorRuntimeHours\":\"" ("string")
            n4022 = local read "model num"() -> (w5224:string[])
            n4023 = local read "Sensor name"() -> (w5243:string[])
            n4024 = local read "run"() -> (w5214:string[])
            n4025 = local read "SENSOR TIME"() -> (w5170:dbl)
            n4026 = local read "out"() -> (w5163:string[])
            n4027 = local read "Total No. of Tests"() -> (w5168:dbl)
            n4028 = Select(t=60.0, s="Run test 3", f=3600.0) -> (s? t:f=w5178:dbl)
            n4029 = Index Array(array=w5224, index #1=1 ("index")) -> (element #1=w5223:string, element #2=w5222:string, element #3=w5221:string, element #4=w5220:string, element #5=w5219:string, element #6=w5218:string)  [unwired: 5 in]
            n4030 = Index Array(array=w5214, index #1=1 ("index")) -> (element #1=w5213:string, element #2=w5212:string, element #3=w5211:string, element #4=w5210:string, element #5=w5209:string, element #6=w5208:string)  [unwired: 5 in]
            n4031 = Index Array(array=w5243, index #1=1 ("index")) -> (element #1=w5242:string, element #2=w5241:string, element #3=w5240:string, element #4=w5239:string, element #5=w5229:string, element #6=w5228:string)  [unwired: 5 in]
            n4032 = Index Array(array=w5163, index #1=1 ("index")) -> (element #1=w5195:string, element #2=w5194:string, element #3=w5193:string, element #4=w5192:string, element #5=w5191:string, element #6=w5190:string)  [unwired: 5 in]
            n4033 = local read "SEN.RUN HRS"() -> (w5166:dbl)
            n4034 = Divide(x=w5170, y=w5178) -> (x/y=w5177:dbl)
            n4035 = Increment(x=w5177) -> (x+1=w5173:dbl)
            n4036 = Number To Decimal String(number=w5173) -> (decimal integer string=→"run hrs":string)  [unwired: 1 in]
            n4037 = Divide(x=w5166, y=3600.0 ("f")) -> (x/y=w5161:dbl)
            n4038 = Round To Nearest(number=w5161) -> (nearest integer value=w5159:dbl)
            n4039 = Number To Decimal String(number=w5159) -> (decimal integer string=w5160:string)  [unwired: 1 in]
            n4040 = Number To Decimal String(number=w5168) -> (decimal integer string=w5169:string)  [unwired: 1 in]
            n4041 = local read "Model No"() -> (w5174:string)
            n4042 = local read "UUID"() -> (w5269:string)
            n4043 = local read "Serial No"() -> (w5273:string)
            n4044 = local read "Secret Key"() -> (w5274:string)
            n4045 = Concatenate Strings("\",\"MachineSerialNumber\":\"" ("string"), w5273) -> (w5277:string)
            n4046 = Concatenate Strings("\",\"ModelNumber\":\"" ("string"), w5174) -> (w5175:string)
            n4047 = Concatenate Strings("\",\"MachineRuntimeHours\":\"" ("string"), w5160) -> (w5278:string)
            n4048 = Concatenate Strings("\",\"MachineRuntimeCycles\":\"", w5169) -> (w5271:string)
            n4049 = Concatenate Strings(w5227, w5223) -> (w5257:string)
            n4050 = Concatenate Strings(w5226, w5213) -> (w5258:string)
            n4051 = Concatenate Strings(w5225, w5195) -> (w5256:string)
            n4052 = Concatenate Strings(w5277, w5175, w5278, w5271) -> (w5280:string)
            n4053 = Concatenate Strings(w5227, w5222) -> (w5254:string)
            n4054 = Concatenate Strings(w5226, w5212) -> (w5253:string)
            n4055 = Concatenate Strings(w5225, w5194) -> (w5255:string)
            n4056 = Concatenate Strings(w5227, w5221) -> (w5249:string)
            n4057 = Concatenate Strings(w5226, w5211) -> (w5250:string)
            n4058 = Concatenate Strings(w5225, w5193) -> (w5248:string)
            n4059 = Concatenate Strings(w5227, w5220) -> (w5246:string)
            n4060 = Concatenate Strings(w5226, w5210) -> (w5245:string)
            n4061 = Concatenate Strings(w5225, w5192) -> (w5247:string)
            n4062 = Concatenate Strings(w5257, w5258, w5256) -> (w5259:string)
            n4063 = Concatenate Strings(w5227, w5219) -> (w5236:string)
            n4064 = Concatenate Strings(w5226, w5209) -> (w5237:string)
            n4065 = Concatenate Strings(w5227, w5218) -> (w5233:string)
            n4066 = Concatenate Strings(w5226, w5208) -> (w5232:string)
            n4067 = Concatenate Strings(w5225, w5191) -> (w5235:string)
            n4068 = Concatenate Strings(w5225, w5190) -> (w5234:string)
            n4069 = Concatenate Strings("{\"SecretKey\":\"", w5274, w5280, "\",\"UUID\" : \"", w5269, "\",\"SensorInformation\":", "[{" ("string")) -> (w5207:string)
            n4070 = Concatenate Strings(w5254, w5253, w5255) -> (w5252:string)
            n4071 = Concatenate Strings(w5249, w5250, w5248) -> (w5251:string)
            n4072 = Concatenate Strings(w5246, w5245, w5247) -> (w5244:string)
            n4073 = Concatenate Strings(w5236, w5237, w5235) -> (w5238:string)
            n4074 = Concatenate Strings(w5233, w5232, w5234) -> (w5231:string)
            n4075 = Concatenate Strings(w5230, w5242, w5259, w5200) -> (w5206:string)
            n4076 = Concatenate Strings(w5230, w5241, w5252, w5200) -> (w5205:string)
            n4077 = Concatenate Strings(w5230, w5240, w5251, w5200) -> (w5204:string)
            n4078 = Concatenate Strings(w5230, w5239, w5244, w5200) -> (w5203:string)
            n4079 = Concatenate Strings(w5230, w5229, w5238, w5200) -> (w5202:string)
            n4080 = Concatenate Strings(w5230, w5228, w5231, "\"}" ("string")) -> (w5201:string)
            n4081 = Concatenate Strings(w5207, w5206, w5205, w5204, w5203, w5202, w5201, "]}" ("string")) -> (w5198:string)
            n4082 = local read "SEN.RUN HRS"() -> (w5165:dbl)
            n4083 = disable-structure shown="Disabled" {
              frame Disabled {
                n4084 = local read "state"() -> (w5284:string[])
                n4085 = Delete From Array(array=w5284, index=0) -> (array with subset deleted=w5282:string[])  [unwired: 1 in, 1 out]
                n4086 = for {
                  N: 6 -> [_]
                  tunnel: w5282 -> [w5295] mode=indexing
                  tunnel: [w5294] -> w5281 mode=indexing
                  n4087 = Equal?(x=w5295, y="Warning") -> (x = y?=w5291:bool)
                  n4088 = Equal?(x=w5295, y="Healthy") -> (x = y?=w5288:bool)
                  n4089 = Select(t="2" ("y"), s=w5291, f="3" ("y")) -> (s? t:f=w5286:string)
                  n4090 = Select(t="1" ("y"), s=w5288, f=w5286) -> (s? t:f=w5294:string)
                }
                "state1" <- w5281
              }
              frame Enabled {
              }
            }
            n4091 = stacked-sequence {
              tunnel: w5198 -> [w5306 _ _]
              tunnel: [_ _ w5322] -> _
              frame #0 {
                (unwired) FALSE ("convert eol (F)")
                w5308 = enum16{"start", "end", "current"}."start" ("pos mode (0:2)")
                n4092 = local read "Path"() -> (w5302:path)
                n4093 = Path To String(path=w5302) -> (string=w5314:string)
                n4094 = Concatenate Strings(w5314, "\\", "Sensor File Name") -> (w5315:string)
                n4095 = local write "standard output 2"(" ") -> ()
                n4096 = String To Path(string=w5315) -> (path=w5305:path)
                n4097 = call <vilib>:"Open_Create_Replace File.vi"("advisory dialog? (display:T)"=FALSE, "function (open:0)"=T28."create or replace", "file path"=w5305) -> ("error out"=w5318:errorcluster, "refnum"=w5317:refnum<file>)  [unwired: 5 in, 2 out]
                n4098 = Set File Position(refnum=w5317, from (0:start)=w5308, error in=w5318) -> (refnum out=w5298:refnum<file>, error out=w5297:errorcluster)  [unwired: 1 in]
                n4099 = Write to Binary File(file (use dialog)=w5298, data=" ", error in=w5297, 5:FALSE ("prepend array or string size? (T)")) -> (refnum out=w5309:refnum<file>, error out=w5310:errorcluster)  [unwired: 2 in, 1 out]
                n4100 = Set File Position(offset (in bytes) (0)=w5308, refnum=w5309, error in=w5310) -> (refnum out=w5301:refnum<file>, error out=w5300:errorcluster)  [unwired: 1 in]
                n4101 = Write to Binary File(file (use dialog)=w5301, data=w5306, error in=w5300, 5:FALSE ("prepend array or string size? (T)")) -> (error out=w5304:errorcluster)  [unwired: 2 in, 2 out]
                n4102 = flat-sequence {
                  tunnel: w5305 -> [w5320]
                  tunnel: w5304 -> [_]
                  frame #0 {
                    n4103 = call <vilib>:"Read Characters From File.vi"("file path (dialog if empty)"=w5320) -> ("character string"=→"Sensor Health JSON string":string)  [unwired: 5 in, 3 out]
                  }
                }
                "SinglePoint  2" <- w5306
              }
              frame #1 {
              }
              frame #2 {
                (unwired) "\"Stored\": true" ("string")
                n4104 = call <vilib>:"System Exec.vi"("run minimized? (F)"=TRUE, "wait until completion? (T)"=TRUE, "working directory"=path "C:/LAB-IQ-NXT", "command line"="C:\\LAB-IQ-NXT\\JPostH.bat") -> ("standard error"=→"Respose From Server 2":string, "standard output"=w5325:string)  [unwired: 4 in, 2 out]
                "standard output 2" <- w5325
                n4105 = Match Pattern(string=w5325, regular expression="JSONH Check String") -> (match substring=w5323:string, offset past match=w5322:i32)  [unwired: 1 in, 2 out]
                n4106 = Equal?(x=w5323, y="JSONH Check String") -> (x = y?=→"Upload \nConfirmed 2":bool)
              }
            }
            n4107 = Divide(x=w5165, y=3600.0 ("f")) -> (x/y=w5158:dbl)
            n4108 = local read "run time"() -> (w5215:string[])
            n4109 = Round To Nearest(number=w5158) -> (nearest integer value=w5157:dbl)
            n4110 = Number To Decimal String(number=w5157) -> (decimal integer string=w5156:string)  [unwired: 1 in]
            n4111 = Index Array(array="Sensor Information", index (col) #1=0 ("disabled index (col)"), index (col) #2=1 ("index (col)"), index (col) #3=2 ("index (col)"), index (col) #4=3 ("index (col)")) -> (element #1=→"Sensor name":string[], element #2=→"model num":string[], element #3=→"run time":string[], element #4=→"state":string[])  [unwired: 4 in]
            n4112 = Insert Into Array(array=w5215, index=1, new element #1=w5156, new element #2=w5156, new element #3=w5156, new element #4=w5156, new element #5=w5156, new element #6=w5156) -> (w5180:string[])
            "run" <- w5180
            n4113 = local read "out"() -> (w5162:string[])
            n4114 = local read "Sensor Information"() -> (w5182:string[][])
            n4115 = Replace Array Subset(array=w5182, new element #1=w5180, index (col) #1=2 ("disabled index (col)"), new element #2=w5162, index (col) #2=3 ("index (col)")) -> (w5181:string[][])  [unwired: 2 in]
            n4116 = local write "Sensor Information"(w5181) -> ()
          }
        }
        n4117 = case shown="True" w5129 {
          frame False {
          }
          frame True {
            n4118 = Equal?(x="FLAG", y=0.0) -> (x = y?=w5146:bool)
            n4119 = case shown="False" w5146 {
              frame False {
                n4120 = Get Date/Time In Seconds() -> (seconds since 1Jan1904=w5152:timestamp)
                n4121 = local read "START 2"() -> (w5150:dbl)
                n4122 = To Double Precision Float(number=w5152) -> (double precision float=w5151:dbl)
                n4123 = Subtract(x=w5151, y=w5150) -> (x-y=→"SENSOR TIME  2":dbl)
              }
              frame True {
                n4124 = Get Date/Time In Seconds() -> (seconds since 1Jan1904=w5154:timestamp)
                n4125 = To Double Precision Float(number=w5154) -> (double precision float=→"START 2":dbl)
                n4126 = local write "FLAG"(100.0 ("FLAG")) -> ()
              }
            }
          }
        }
        n4127 = disable-structure shown="Disabled" {
          disable-tunnel: w5132 -> [w5141 _]
          disable-tunnel: [w5140 _] -> w5131
          frame Disabled {
            n4128 = local read "Json St Flg"() -> (w5139:bool)
            n4129 = case shown="True" w5139 {
              tunnel: w5141 -> [w5142 w5144]
              tunnel: [w5142 w5143] -> w5140
              frame False {
              }
              frame True {
                n4130 = Increment(x=w5144) -> (x+1=w5143:dbl)
                "T cycle" <- w5143
                n4131 = local write "Json St Flg"(FALSE ("Json St Flg")) -> ()
              }
            }
          }
          frame Enabled {
          }
        }
        n4132 = local read "Quit"() -> (w5126:bool)
      }
    }
    frame Enabled {
    }
  }
  n4133 = stacked-sequence {
    tunnel: [w5524] -> w35
    frame #0 {
      w5524 = FALSE ("Upload \nConfirmed")
      n4134 = local write "Upload \nConfirmed"(w5524) -> ()
      n4135 = local write "St Str"("") -> ()
    }
  }
  n4136 = disable-structure shown="Disabled" {
    disable-tunnel: w35 -> [w5525 _]
    frame Disabled {
      n4137 = case shown="True" {
        selector: _ -> [_ _]
        tunnel: w5525 -> [_ w5526]
        frame False {
        }
        frame True {
          n4138 = while {
            tunnel: [w5532] -> _
            tunnel: w5526 -> [_]
            i -> [w5532]
            stop <- w5527 stop-if-true
            n4139 = local read "Json End Flg"() -> (w5531:bool)
            n4140 = Wait (ms)(milliseconds to wait=u32 20 ("Refresh Rate (ms)")) -> ()  [unwired: 1 out]
            n4141 = local read "refresh flag"() -> (w5528:bool)
            n4142 = local read "RUN"() -> (w5529:bool)
            n4143 = And(x=w5529, y=w5528) -> (x .and. y?=w5530:bool)
            n4144 = Or(x=w5530, y=w5531) -> (x .or. y?=w5533:bool)
            "AR Led" <- w5533
            n4145 = case shown="True" w5533 {
              frame False {
              }
              frame True {
                w5550 = "\",\""
                n4146 = local read "UUID"() -> (w5548:string)
                n4147 = local write "refresh flag"(FALSE ("refresh flag")) -> ()
                n4148 = local read "time"() -> (w5537:dbl)
                n4149 = Multiply(x=w5537, y=60.0) -> (x*y=w5536:dbl)
                n4150 = Concatenate Strings("UUID\" : \"", w5548, "\"}") -> (w5551:string)
                n4151 = Number To Fractional String(number=w5536, width (-)=i16 10, precision (6)=i16 4) -> (F-format string=w5565:string)  [unwired: 1 in]
                n4152 = Concatenate Strings("{", "\"Time\":\"", w5565, w5550) -> (w5560:string)
                n4153 = stacked-sequence {
                  tunnel: w5550 -> [w5613 w5621 w5628 w5636 w5644 w5653 w5660]
                  tunnel: [w5614 _ _ _ _ _ _] -> w5564
                  tunnel: [_ w5622 _ _ _ _ _] -> w5563
                  tunnel: [_ _ w5629 _ _ _ _] -> w5562
                  tunnel: [_ _ _ w5638 _ _ _] -> w5561
                  tunnel: w5551 -> [_ _ _ _ _ _ w5671]
                  tunnel: [_ _ _ _ _ _ w5670] -> w5547
                  tunnel: [_ _ _ _ _ w5650 _] -> w5546
                  tunnel: [_ _ _ _ w5643 _ _] -> w5545
                  frame #0 {
                    n4154 = local read "NORMAL LOAD"() -> (w5612:dbl)
                    n4155 = Number To Fractional String(number=w5612, width (-)=i16 10, precision (6)=i16 4) -> (F-format string=w5615:string)  [unwired: 1 in]
                    n4156 = Concatenate Strings("NormalLoad\":\"", w5615, w5613) -> (w5614:string)
                  }
                  frame #1 {
                    n4157 = local read "Temp"() -> (w5620:dbl)
                    n4158 = Number To Fractional String(number=w5620, width (-)=i16 10, precision (6)=i16 4) -> (F-format string=w5623:string)  [unwired: 1 in]
                    n4159 = Concatenate Strings("Temperature\":\"", w5623, w5621) -> (w5622:string)
                  }
                  frame #2 {
                    n4160 = local read "cof"() -> (w5626:dbl)
